vi "Read.vi"(8 "error out":errorcluster caption="error in", 10 "Command":T1={"Index"="``", "Sub-Index"="\u0000", "Data-Size (in Byte)"=1} {"Data-Size (in Byte)" min=1 max=4 step=1 format="%x"}, 11 "ComPort In":refnum<visa-resource-name>) -> (0 "error out 2":errorcluster caption="error out", 2 "Answer":i32, 3 "ComPort Out":refnum<visa-resource-name>)   [LabVIEW 2021, in "Nanotech PDC-4.lvlib"]
uses:
  Nanotech PDC-4.lvlib
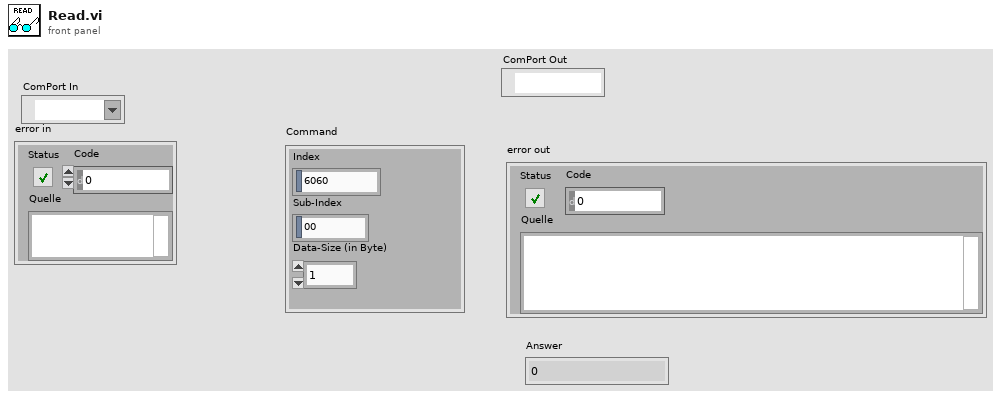
[diagram p1: front panel]
types:
  T1 = cluster{"Index":string, "Sub-Index":string, "Data-Size (in Byte)":u8}
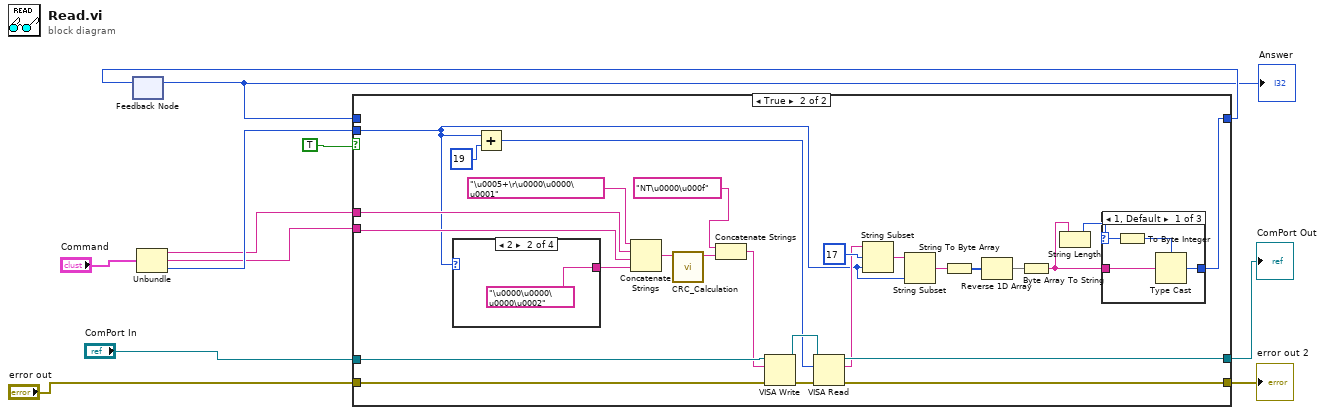
[diagram p0: block diagram]
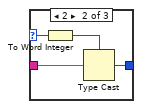
[diagram p3: hidden frame]
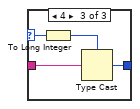
[diagram p4: hidden frame]
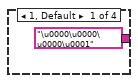
[diagram p5: hidden frame]
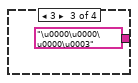
[diagram p6: hidden frame]
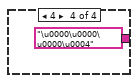
[diagram p7: hidden frame]
diagram:
  n1 = feedback #1() -> (w9:i32)  [unwired: 1 in]
  "Answer" <- w9
  n2 = Unbundle("Command") -> ("Index"=w4:string, "Sub-Index"=w3:string, "Data-Size (in Byte)"=w5:u8)
  n3 = case shown="True" TRUE {
    tunnel: "ComPort In" -> [w13 w37]
    tunnel: "error out" -> [w14 w36]
    tunnel: [w14 w33] -> w11
    tunnel: w5 -> [_ w16]
    tunnel: w4 -> [_ w32]
    tunnel: w3 -> [_ w31]
    tunnel: [w13 w28] -> w7
    tunnel: [w12 w18] -> w10
    tunnel: w9 -> [w12 _]
    frame False {
    }
    frame True {
      n4 = case shown="2" w16 {
        tunnel: ["\u0000\u0000\u0000\u0001" ("Hexadecimal Input String 4") "\u0000\u0000\u0000\u0002" ("Hexadecimal Input String 4") "\u0000\u0000\u0000\u0003" ("Hexadecimal Input String 4") "\u0000\u0000\u0000\u0004" ("Hexadecimal Input String 4")] -> w27
        frame 1, Default {
        }
        frame 2 {
        }
        frame 3 {
        }
        frame 4 {
        }
      }
      n5 = Add(x=w16, y=u32 19 ("byte count")) -> (x+y=w29:u32)
      n6 = Concatenate Strings("\u0005+\r\u0000\u0000\u0001" ("Hexadecimal Input String 4"), w32, w31, w27) -> (w35:string)
      n7 = call "CRC_Calculation.vi"("CMD"=w35) -> ("CMD + CRC"=w34:string)  [unwired: 10 in]
      n8 = Concatenate Strings("NT\u0000\u000f" ("Hexadecimal Input String 4"), w34) -> (w26:string)
      n9 = VISA Write(VISA resource name=w37, write buffer=w26, error in (no error)=w36) -> (VISA resource name out=w39:refnum<visa-resource-name>, error out=w40:errorcluster)  [unwired: 1 out]
      n10 = VISA Read(VISA resource name=w39, byte count=w29, error in (no error)=w40) -> (VISA resource name out=w28:refnum<visa-resource-name>, read buffer=w17:string, error out=w33:errorcluster)  [unwired: 1 out]
      n11 = String Subset(string=w17, offset (0)=u8 17 ("x"), length (rest)=w16) -> (substring=w20:string)
      n12 = String Subset(string=w20, length (rest)=w16) -> (substring=w23:string)  [unwired: 1 in]
      n13 = String To Byte Array(string=w23) -> (unsigned byte array=w22:u8[])
      n14 = Reverse 1D Array(array=w22) -> (reversed array=w21:u8[])
      n15 = Byte Array To String(unsigned byte array=w21) -> (string=w25:string)
      n16 = String Length(string=w25) -> (length=w24:i32)
      n17 = case shown="1, Default" w24 {
        selector: w24 -> [w44 w48 w52]
        tunnel: w25 -> [w41 w46 w51]
        tunnel: [w42 w45 w50] -> w18
        frame 1, Default {
          n18 = To Byte Integer(number=w44) -> (8bit integer=w43:i8)
          n19 = Type Cast(type=w43, x=w41) -> (*(type *) &x=w42:i8)
        }
        frame 2 {
          n20 = To Word Integer(number=w48) -> (16bit integer=w47:i16)
          n21 = Type Cast(type=w47, x=w46) -> (*(type *) &x=w45:i16)
        }
        frame 4 {
          n22 = To Long Integer(number=w52) -> (32bit integer=w49:i32)
          n23 = Type Cast(type=w49, x=w51) -> (*(type *) &x=w50:i32)
        }
      }
    }
  }
  "error out 2" <- w11
  "ComPort Out" <- w7
  n24 = feedback-in #1(w10) -> ()
